vi "PH_Beamline.color MA BL.vi"(0 "i ref in":refnum<vi>, 2 "Color State MA Input":i32, 5 "error in (no error)":errorcluster) -> (14 "i ref out":refnum<vi>, 16 "Color State MA Exit to MAS":i32, 17 "Color State MA Exit to Booster":i32, 19 "error out":errorcluster)   [LabVIEW 2014, in "PH_Beamline.lvlib"]
doc: "This Vi colors the MainAmp beamline elements."
uses:
  PH_Beamline.lvlib
  PH_StatusHandler/PH_StatusHandler.Status.ctl
  PH_Common/PH_Common.lvlib
  PH_BL-Master/PH_BL-Master.lvlib
  PH_StatusHandler/PH_StatusHandler.lvlib
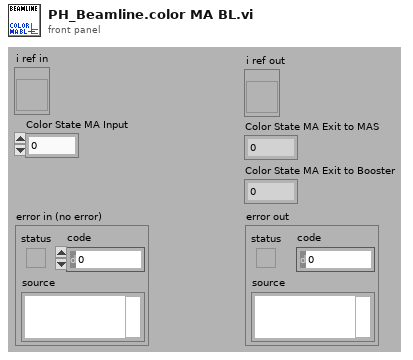
[diagram p1: front panel]
types:
  T1 = typedef "PH_StatusHandler.lvlib/PH_StatusHandler.Status.ctl" = i16
  T2 = typedef "PH_Beamline.lvlib/PH_Beamline.i attribute.ctl" = cluster{"GUI Refs":cluster{"PA ok":refnum<vi>, "MA ok":refnum<vi>, "fs FE ok":refnum<vi>, "ns FE ok":refnum<vi>, "PA ED ok":refnum<vi>, "MAS ok":refnum<vi>, "Booster ok":refnum<vi>, "Mirrortower ok":refnum<vi>, "In.-Box ok":refnum<vi>, "Compressor ok":refnum<vi>, "Experiment LB ok":refnum<vi>, "Experiment LL ok":refnum<vi>, "PHELIX_Beckhoff_Watchdog":refnum<vi>, "Shutters closed":refnum<vi>, "uOPA ok":refnum<vi>, "Vacuum no shotcond Comp LB":refnum<vi>}, "Refs BL MA":refnum<vi>[], "Refs BL MA-IB":refnum<vi>[], "Refs BL fs":refnum<vi>[], "Refs BL PA ED":refnum<vi>[], "Refs BL MAS":refnum<vi>[], "Refs BL Boo":refnum<vi>[], "Refs BL ns":refnum<vi>[], "Refs BL Mirrortower":refnum<vi>[], "Refs BL Compressor":refnum<vi>[], "Refs BL Exp LB":refnum<vi>[], "Radiation Safety":cluster{"Exp Laserbay":cluster{"Ref Op Mode":refnum<vi>, "Ref Laserbay evacuated":refnum<vi>, "Tagname LB evacuated":string, "Shot Mode":T3, "Laserbay evacuated?":i32, "Tagname HV room locked":string, "HV room locked?":i32, "Ref HV room locked":refnum<vi>, "Tagname bridged?":string, "Ref Bridge":refnum<vi>, "I<1E18W/cm²":bool}, "Exp Laserlab":cluster{"Ref Op Mode":refnum<vi>, "Ref Laserlab evacuated":refnum<vi>, "Tagname LL evacuated":string, "Shot Mode":T3, "Laserlab evacuated?":i32, "Tagname bridged?":string, "Ref Bridge":refnum<vi>, "I<1E18W/cm²":bool}}, "Refs BL LL":refnum<vi>[], "PP Igni Heating GUI Refs":refnum<vi>[], "PP Igni Heating Tagnames ":string[], "Refs BL PA":cluster{"undelayed Line before Shutter":refnum<vi>[], "undelayed Line after Shutter":refnum<vi>[], "before Bypass":refnum<vi>[], "delayed Line before Shutter":refnum<vi>[], "delayed Line after Shutter":refnum<vi>[], "before Shutter Input":refnum<vi>[], "after Shutter Input":refnum<vi>[], "Bypass":refnum<vi>[], "before Shutter Exit":refnum<vi>[], "after Shutter Exit":refnum<vi>[], "to MA":refnum<vi>[], "to Lab":refnum<vi>[]}, "BL":cluster{"YLF_BL_Status":i32, "fs_BL_Status":i32, "fs_YLF_BL_Status":i32, "ns_BL_Status":i32, "PA_Input_BL_Status":i32, "PA_UnDelay_BL_Status":i32, "PA_Delay_BL_Status":i32, "PA_BL_Status":i32, "PA_Bypass_BL_Status":i32, "PA_Exit_BL_Status":i32, "PA_LL_BL_Status":i32, "LL_BL_Status":i32, "PA_MA_BL_Status":i32, "MA_Exit_BL_Status":i32, "MA_Z6_BL_Status":i32, "Z6_BL_Status":i32, "MA_LB_BL_Status":i32, "LB_TB2_BL_Status":i32, "PA_before_Bypass_BL_Status":i32, "LB_TB3_BL_Status":i32}, "State Subsystems":cluster{"PA":bool, "MA":bool, "ns FE":bool, "fs FE":bool, "PA ED":bool, "In.-Box":bool, "MAS":bool, "Booster":bool, "Mirrortower":bool, "Compressor":bool, "Experiment LB":bool, "Experiment LL":bool, "uOPA":bool}, "Status Subscriber Information":T4, "Refs BL uOPA":refnum<vi>[], "PA_Input_2_Beam_6PWpGUI not linked?":bool, "PA_Input_Delay_6PGUI not linked?":bool, "Settings":T7}
  T3 = typedef "PH_Beamline.lvlib/PH_Beamline.Operation Mode.ctl" = i32
  T4 = typedef "PH_Beamline.lvlib/PH_Beamline.Status Subscriber Information.ctl" = cluster{"fs Swich YLF":T5, "fs Exit Shutter":T5, "ns Exit Shutter":T5, "PA Input Shutter":T5, "PA PC WP":T5, "PA PC WP 2":T5, "PA Bypass In":T5, "PA Bypass Out":T5, "PA CH 1":T5, "PA delayed":T5, "PA non delayed":T5, "PA Exit Shutter":T5, "PA Switch Lab":T5, "PA Bridge CH Input MA":T5, "MA Diffusor IB":T5, "MA IB Ready":T5, "MA CH 1":T5, "MA CH 2":T5, "MA CH 3":T5, "MA CH 4":T5, "MA Shutter Align Cam":T5, "MA Position MM5":T5, "Calorimeter Switch":T5, "BL Z6 CH 9":T5, "BL Z6 Beamdump":T5, "BL Z6 Shutter":T5, "COS Sensitivity Switch":T5, "Exp LB Shutter":T5, "Exp LB TB 2":T5, "Exp LB TB 3":T5, "PA LL Input CH":T5, "PA LL Output CH":T5, "LL Comp Input Shutter":T5, "LL Comp Output Shutter":T5, "LL Comp FF Shutter":T5, "Exp LL Shutter":T5, "MA IM In IB":T5, "MA IM Out IB":T5, "MA DB In IB":T5, "MA DB Out IB":T5, "Exp LB Shutter Interlock":T5, "Exp LL Shutter Interlock":T5, "MM1 Force Sensor":T5}
  T5 = typedef "PH_BL-Master.lvlib/PH_BL-Master.Status Subscriber Information.ctl" = cluster{"Index of element":i32, "Attributeset":T6}
  T6 = typedef "PH_BL-Master.lvlib/PH_BL-Master.Attribute Set.ctl" = enum16{"Boolean Status Service Subscriber", "Picture Status Service Subscriber"}
  T7 = typedef "PH_Beamline_Chief.lvlib/PH_Beamline_Chief.Settings.ctl" = cluster{"PA Doublepass Mode":bool, "Compressor Vaccuum LB not relevant":bool, "Windowshutter TB2 not relevant":bool, "Windowshutter TB3 not relevant":bool}
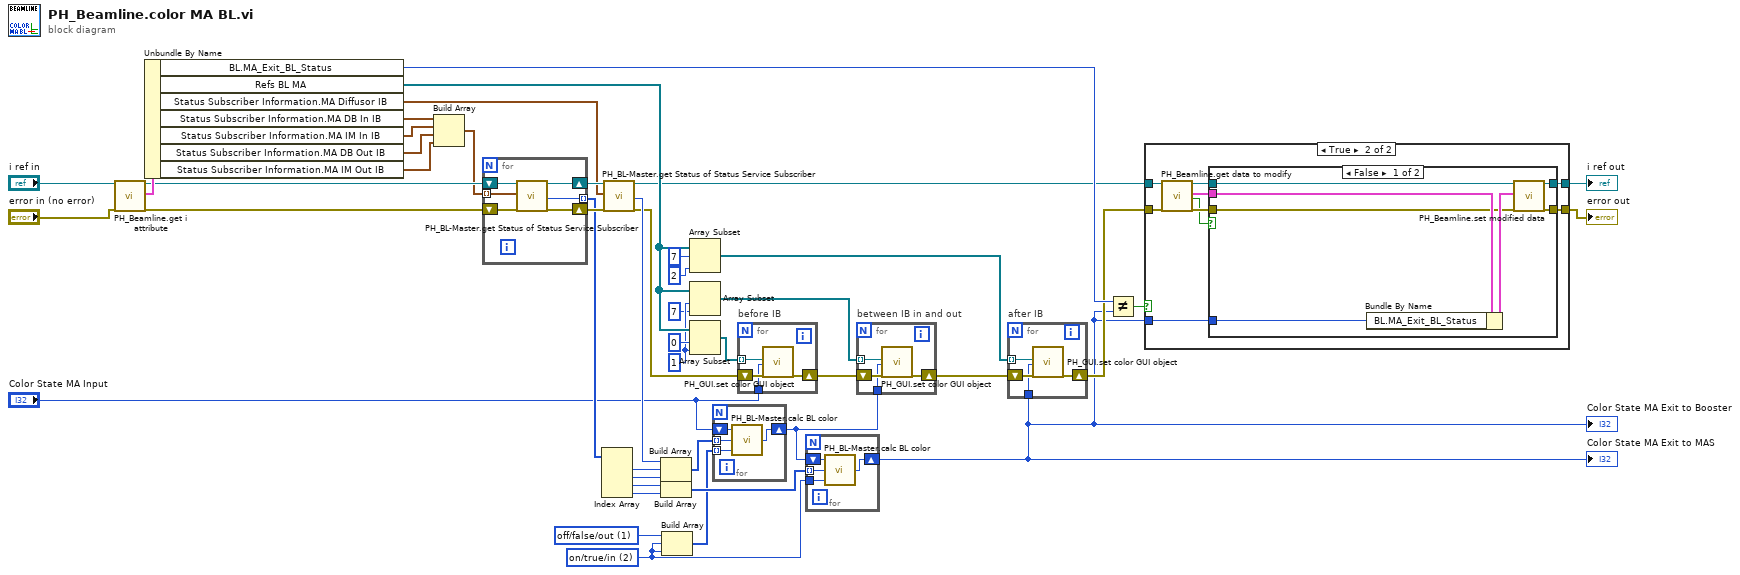
[diagram p0: block diagram]
diagram:
  w21 = T1 1 items=["no info", "off/false/out", "on/true/in", "Failure", "Alarm", "Status 1", "Status 2", "Status 3"] ("State for \"2\" (on) of ABLE (off/false/out)")
  w20 = T1 2 items=["no info", "off/false/out", "on/true/in", "Failure", "Alarm", "Status 1", "Status 2", "Status 3"] ("State for \"2\" (on) of ABLE (off/false/out)")
  w37 = 1 ("length")
  n1 = call "PH_Beamline.get i attribute.vi"("i ref in"="i ref in", "error in (no error)"="error in (no error)") -> ("i ref out"=w9:refnum<vi>, "i attribute"=w45:T2, "error out"=w8:errorcluster)  [unwired: 15 in]
  n2 = Unbundle By Name(w45) -> ("BL.MA_Exit_BL_Status"=w16:i32, "Refs BL MA"=w38:refnum<vi>[], "Status Subscriber Information.MA Diffusor IB"=w10:T5, "Status Subscriber Information.MA DB In IB"=w5:T5, "Status Subscriber Information.MA IM In IB"=w4:T5, "Status Subscriber Information.MA DB Out IB"=w3:T5, "Status Subscriber Information.MA IM Out IB"=w2:T5)
  n3 = Build Array(w5, w4, w3, w2) -> (w1:T5[])
  n4 = for {
    tunnel: w1 -> [w50] mode=indexing
    tunnel: [w47] -> w31 mode=indexing
    shift-right: [w49] -> w44
    shift-left: w9 -> [w46]
    shift-right: [w48] -> w43
    shift-left: w8 -> [w51]
    n5 = call "PH_BL-Master.get Status of Status Service Subscriber.vi"("i ref in"=w46, "Wanted Status Subscriber Information"=w50, "error in (no error)"=w51) -> ("i ref out"=w49:refnum<vi>, "Status"=w47:T1, "error out"=w48:errorcluster)  [unwired: 11 in, 3 out]
  }
  n6 = Index Array(array=w31) -> (element #1=w27:T1, element #2=w26:T1, element #3=w25:T1, element #4=w24:T1)  [unwired: 4 in]
  n7 = call "PH_BL-Master.get Status of Status Service Subscriber.vi"("i ref in"=w44, "Wanted Status Subscriber Information"=w10, "error in (no error)"=w43) -> ("i ref out"=w7:refnum<vi>, "Status"=w29:T1, "error out"=w6:errorcluster)  [unwired: 11 in, 3 out]
  n8 = Build Array(w29, w27, w26) -> (w23:T1[])
  n9 = Build Array(w25, w24) -> (w22:T1[])
  n10 = Build Array(w21, w20, w20) -> (w19:T1[])
  n11 = Array Subset(array=w38, index=7, length=2) -> (w33:refnum<vi>[])
  n12 = Array Subset(array=w38, index=w37, length=7) -> (w32:refnum<vi>[])
  n13 = Array Subset(array=w38, index=0, length=w37) -> (w42:refnum<vi>[])
  n14 = for {
    tunnel: w23 -> [w52] mode=indexing
    tunnel: w19 -> [w54] mode=indexing
    shift-right: [w53] -> w30
    shift-left: "Color State MA Input" -> [w55]
    n15 = call "PH_BL-Master.calc BL color.vi"("State for \"2\" (on) of ABLE (off/false/out)"=w54, "State ABLE"=w52, "State before ABLE"=w55) -> ("State after ABLE"=w53:i32)
  }
  n16 = for "before IB" {
    tunnel: w42 -> [w59] mode=indexing
    shift-right: [w57] -> w39
    shift-left: w6 -> [w58]
    tunnel: "Color State MA Input" -> [w56]
    n17 = call "PH_GUI.set color GUI object.vi"("GUI object Ref"=w59, "State"=w56, "error in (no error)"=w58) -> ("error out"=w57:errorcluster)  [unwired: 16 in]
  }
  n18 = for {
    tunnel: w22 -> [w60] mode=indexing
    tunnel: w20 -> [w62]
    shift-right: [w61] -> w13
    shift-left: w30 -> [w63]
    n19 = call "PH_BL-Master.calc BL color.vi"("State for \"2\" (on) of ABLE (off/false/out)"=w62, "State ABLE"=w60, "State before ABLE"=w63) -> ("State after ABLE"=w61:i32)
  }
  "Color State MA Exit to Booster" <- w13
  "Color State MA Exit to MAS" <- w13
  n20 = for "between IB in and out" {
    tunnel: w32 -> [w67] mode=indexing
    shift-right: [w65] -> w40
    shift-left: w39 -> [w66]
    tunnel: w30 -> [w64]
    n21 = call "PH_GUI.set color GUI object.vi"("GUI object Ref"=w67, "State"=w64, "error in (no error)"=w66) -> ("error out"=w65:errorcluster)  [unwired: 16 in]
  }
  n22 = for "after IB" {
    tunnel: w33 -> [w71] mode=indexing
    shift-right: [w69] -> w15
    shift-left: w40 -> [w70]
    tunnel: w13 -> [w68]
    n23 = call "PH_GUI.set color GUI object.vi"("GUI object Ref"=w71, "State"=w68, "error in (no error)"=w70) -> ("error out"=w69:errorcluster)  [unwired: 16 in]
  }
  n24 = Not Equal?(x=w16, y=w13) -> (x != y?=w18:bool)
  n25 = case shown="True" w18 {
    tunnel: w7 -> [w73 w78]
    tunnel: [w73 w77] -> w17
    tunnel: w15 -> [w72 w76]
    tunnel: [w72 w75] -> w14
    tunnel: w13 -> [_ w74]
    frame False {
    }
    frame True {
      n26 = call "PH_Beamline.get data to modify.vi"("i ref in"=w78, "error in (no error)"=w76) -> ("i ref out"=w81:refnum<vi>, "i attribute"=w79:T2, "timed out"=w80:bool, "error out"=w82:errorcluster)  [unwired: 14 in]
      n27 = case shown="False" w80 {
        tunnel: w82 -> [w83 w90]
        tunnel: w81 -> [w89 w91]
        tunnel: [w88 w90] -> w75
        tunnel: [w87 w91] -> w77
        tunnel: w79 -> [w84 _]
        tunnel: w74 -> [w85 _]
        frame False {
          n28 = Bundle By Name(cluster=w84, "BL.MA_Exit_BL_Status"=w85) -> (w86:T2)
          n29 = call "PH_Beamline.set modified data.vi"("i ref in"=w89, "i attribute"=w86, "error in (no error)"=w83) -> ("i ref out"=w87:refnum<vi>, "error out"=w88:errorcluster)  [unwired: 15 in]
        }
        frame True {
        }
      }
    }
  }
  "error out" <- w14
  "i ref out" <- w17
